vi "Periodic Tasks.vi"(8 "error in":errorcluster) -> ()   [LabVIEW 2014]
doc: "This VI runs in parallel to other tasks. It can contain as many user-defined periodic loops as you need. These can carry out PID or other sorts of timed response."
uses:
  <vilib>/Rock Robotics/WPI/Joystick/WPI_JoystickGetSetRefNum.vi
  Robot Global Data.vi
  <vilib>/Rock Robotics/Network Tables/SD Write Boolean.vi
  <vilib>/Rock Robotics/Network Tables/SD Write Number.vi
  <vilib>/Rock Robotics/WPI/RobotDrive/WPI_RobotDriveGetSetRefNum.vi
  <vilib>/Rock Robotics/WPI/Solenoid/WPI_SolenoidValue.ctl
  <vilib>/Rock Robotics/WPI/Solenoid/WPI_SolenoidSetEnum.vi
panel:
  in  "Stopper Motor Speed Up":dbl(slide)=0.6 min=-1.0 max=1.0 step=0.05 scale=0.0..1.0 scale format="%#.3f"
  in  "Stopper Motor Speed Down":dbl(slide)=0.2 min=-1.0 max=1.0 step=0.05 scale=0.0..1.0 scale format="%#.3f"
  out "Actual Stopper Motor Speed":dbl
  out "Lifting Motor Speed Up":dbl
  out "Mode":bool
  out "Actual Lifting Motor Speed":dbl format="%#_13g"
  out "Trigger Switch Activated":bool=TRUE
  out "Upper Switch Activated":bool=TRUE
  out "Lower Switch Activated":bool=TRUE
  out "Accelerometer Chart":cluster{"X-Axis":dbl, "Y-Axis":dbl}(graph)
  out "X Acceleration":dbl format="%#_13g"
  out "Y Acceleration":dbl format="%#_13g"
  out "Degrees of Rotation":dbl format="%#_13g"
  out "pnumatics button":bool
  out "L":bool
  out "U":bool
  out "T":bool
  out "Running":bool
  out "Direction":bool
  in  "Lifting Motor Speed Down":dbl(slide)=0.2 min=-1.0 max=1.0 step=0.05 scale=0.0..1.0 scale format="%#.3f"
  # "STOPPER\nMOTOR PANEL"
  # "GANTRY LIFT\nMOTOR PANEL"
  # "INDICATORS"
  # "LOGIC"
  # "CONTROLS"
  # "CONTROLS"
  # "INDICATORS"
  # "ACCELEROMETER\nPANEL"
  # "PNEUMATICS\nPANEL"
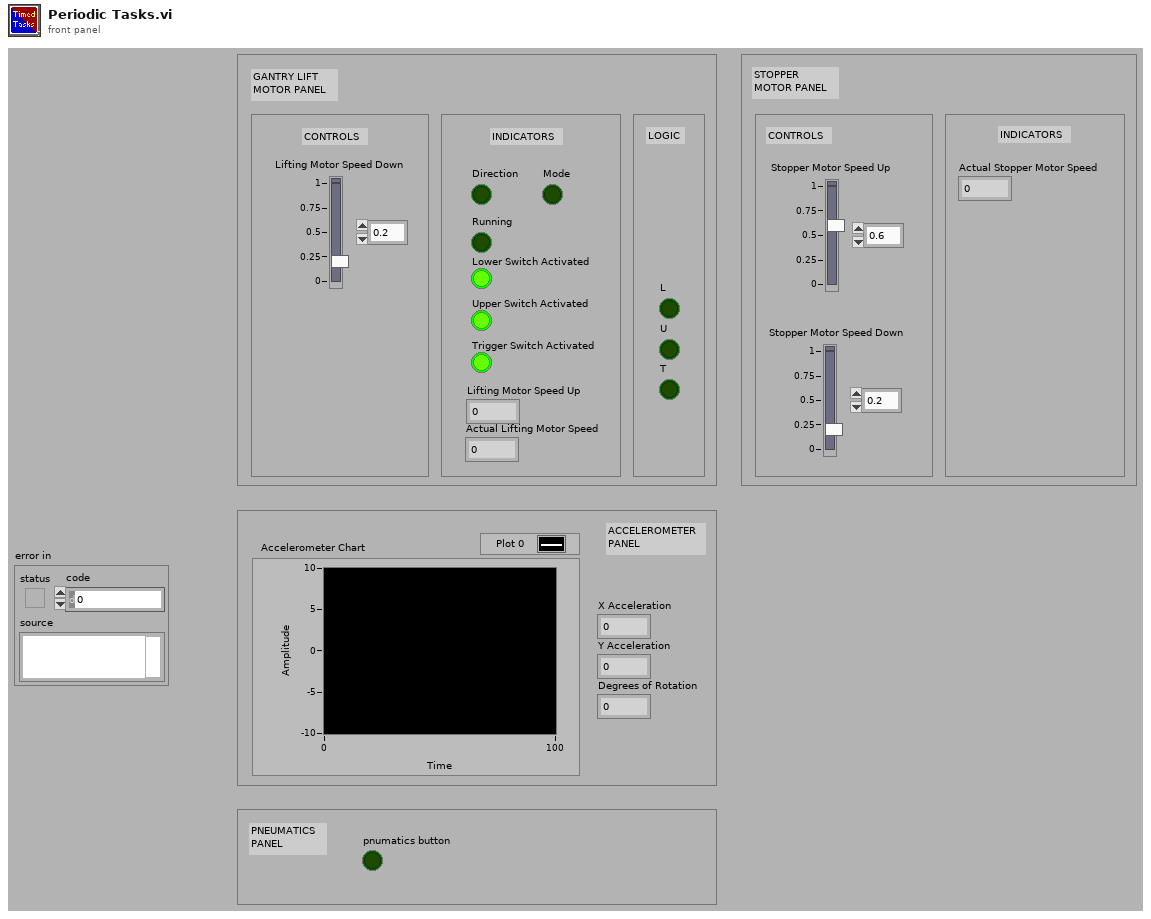
[diagram p1: front panel]
types:
  T1 = typedef "WPI_SolenoidValue.ctl" = enum16{"Off", "On", "Forward", "Reverse"}
  T2 = typedef "WPI_JoystickDevRef.ctl" = cluster{"Device":T3}
  T3 = typedef "WPI_JoystickDeviceEnum.ctl" = enum16{"USB 0", "USB 1", "USB 2", "USB 3", "USB 4", "USB 5"}
  T4 = typedef "WPI_SolenoidDevRef.ctl" = cluster{"DevStatus":errorcluster, "Pneumatics Control Module":u8, "Forward Solenoid Channel":T5, "Reverse Solenoid Channel":T5}
  T5 = typedef "WPI_SolenoidChannel.ctl" = enum8{"Solenoid 0", "Solenoid 1", "Solenoid 2", "Solenoid 3", "Solenoid 4", "Solenoid 5", "Solenoid 6", "Solenoid 7", "Invalid"}
  T6 = cluster{"JoystickDevRef":T2, "SolenoidDevRef":T4}
  T7 = typedef "WPI_AccelerometerDevRef.ctl" = cluster{"DevStatus":errorcluster, "Controller":T8, "Scaling":T9, "Analog Channels":T10, "I2C Bus":T12, "SPI Bus":T13, "Accel Range":T14, "ADXL345 Axes":T15, "Handle":i32, "Device Address":u8, "Accel Type":enum16{"Analog", "ADXL345 I2C", "ADXL345 SPI", "Internal"}}
  T8 = typedef "FPGA_TypedefAnalogModule.ctl" = enum16{"Controller 1"}
  T9 = typedef "WPI_AccelerometerScaling.ctl" = cluster{"Gain (VoltsPerG)":dbl, "Center Voltage":dbl}
  T10 = typedef "WPI_AccelerometerAnalogChannels.ctl" = cluster{"X-Axis":T11, "Y-Axis":T11, "Z-Axis":T11}
  T11 = typedef "FPGA_AIChannel.ctl" = enum8{"AI 0", "AI 1", "AI 2", "AI 3", "AI MXP 0", "AI MXP 1", "AI MXP 2", "AI MXP 3", "Invalid"}
  T12 = typedef "i2c_bus.ctl" = enum16{"I2C On-Board", "I2C MXP", "Invalid"}
  T13 = typedef "spi_bus.ctl" = enum16{"SPI On-Board, CS0", "SPI On-Board, CS1", "SPI On-Board, CS2", "SPI On-Board, CS3", "SPI MXP", "Invalid"}
  T14 = typedef "ADXL345 Range.ctl" = u8
  T15 = typedef "WPI_AccelerometerADXL345 Axes.ctl" = cluster{"X-Axis":bool, "Y-Axis":bool, "Z-Axis":bool}
  T16 = cluster{"X-Axis":dbl, "Y-Axis":dbl, "Z-Axis":dbl}
  T17 = typedef "WPI_MotorControlDeviceRef.ctl" = cluster{"DeviceStatus":errorcluster, "Type":T18, "PWM":cluster{"Controller":T19, "PWM Channel":T20, "DeadBand":T21}, "CAN":cluster{"Device Number":u8, "Control Mode":T22, "Semaphore":T23, "Max Vout":dbl, "TalonSRX Control Mode":T24}, "Invert":bool, "TransformRef":T25, "InvTransformRef":T25}
  T18 = typedef "WPI_MotorControlType.ctl" = enum16{"PWM", "CAN", "CANTalonSRX"}
  T19 = typedef "FPGA_TypedefDigitalModule.ctl" = enum16{"Controller 1"}
  T20 = typedef "FPGA_DIOPWMChannel.ctl" = enum8{"PWM 0", "PWM 1", "PWM 2", "PWM 3", "PWM 4", "PWM 5", "PWM 6", "PWM 7", "PWM 8", "PWM 9", "PWM MXP 0", "PWM MXP 1", "PWM MXP 2", "PWM MXP 3", "PWM MXP 4", "PWM MXP 5", "PWM MXP 6", "PWM MXP 7", "PWM MXP 8", "PWM MXP 9", "Invalid"}
  T21 = typedef "WPI_PWMDeadband.ctl" = cluster{"Name":string, "maxPositivePwm":i32, "minPositivePwm":i32, "centerPwm":i32, "maxNegativePwm":i32, "minNegativePwm":i32, "angularRange":u16}
  T22 = typedef "WPI_CANJaguar_ControlMode.ctl" = enum8{"Percent VBus", "Current", "Speed", "Position", "Voltage"}
  T23 = typedef "Semaphore RefNum" = refnum<k1>
  T24 = typedef "WPI_CANTalonSRX_APIControlMode.ctl" = enum8{"Percent VBus", "Speed", "Position", "Slave", "Unchanged / Invalid"}
  T25 = typedef "WPI_PWMTransform_ConPane.ctl" = refnum<vi>
  T26 = typedef "WPI_DigitalInputDevRef.ctl" = cluster{"DevStatus":errorcluster, "DIO Channel":T27, "Controller":T19}
  T27 = typedef "FPGA_DIOChannel.ctl" = enum8{"DIO 0", "DIO 1", "DIO 2", "DIO 3", "DIO 4", "DIO 5", "DIO 6", "DIO 7", "DIO 8", "DIO 9", "DIO MXP 0", "DIO MXP 1", "DIO MXP 2", "DIO MXP 3", "DIO MXP 4", "DIO MXP 5", "DIO MXP 6", "DIO MXP 7", "DIO MXP 8", "DIO MXP 9", "DIO MXP 10", "DIO MXP 11", "DIO MXP 12", "DIO MXP 13", "DIO MXP 14", "DIO MXP 15", "Invalid"}
  T28 = cluster{"JoystickDevRef":T2, "MotorControlDevRef":T17}
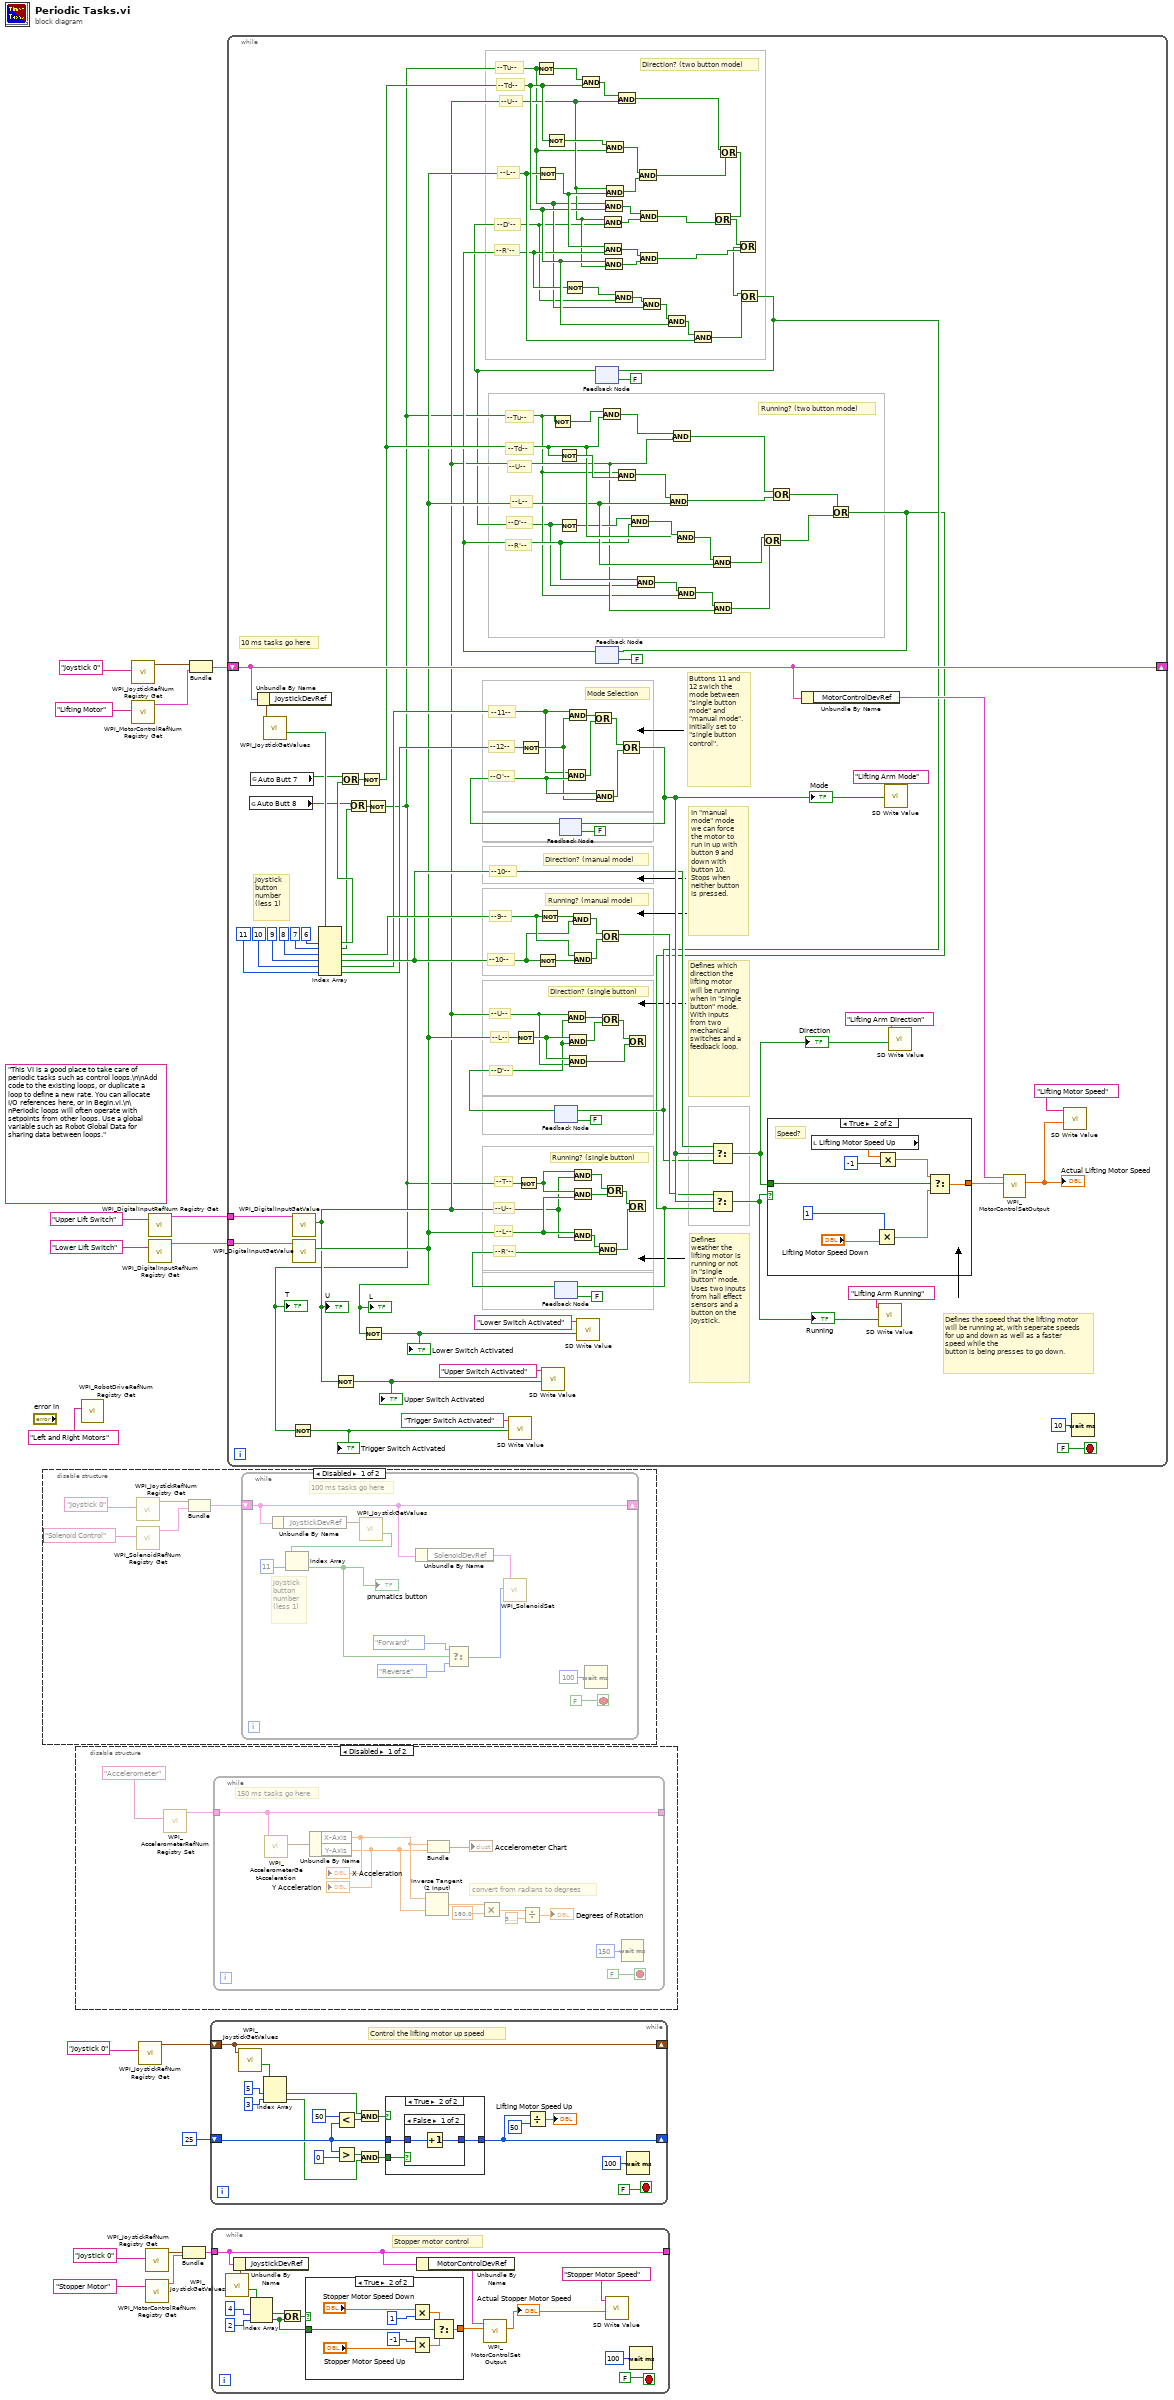
[diagram p0: block diagram]
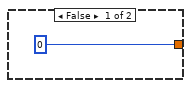
[diagram p2: hidden frame]
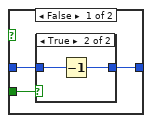
[diagram p3: hidden frame]
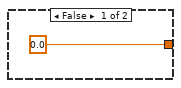
[diagram p8: hidden frame]
diagram:
  (unwired) "This VI is a good place to take care of periodic tasks such as control loops.\n\nAdd code to the existing loops, or duplicate a loop to define a new rate. You can allocate I/O references here, or in Begin.vi.\n\nPeriodic loops will often operate with setpoints from other loops. Use a global variable such as Robot Global Data for sharing data between loops."
  n1 = disable-structure shown="Disabled" {
    frame Disabled {
      n2 = call <vilib>:"WPI_JoystickRefNum Registry Get.vi"("refnum name"="Joystick 0") -> ("JoystickDevRef"=w21:T2)  [unwired: 1 in, 9 out]
      n3 = call <vilib>:"WPI_SolenoidRefNum Registry Get.vi"("refnum name"="Solenoid Control") -> ("SolenoidDevRef"=w20:T4)  [unwired: 9 in, 1 out]
      n4 = Bundle("JoystickDevRef"=w21, "SolenoidDevRef"=w20) -> (w19:T6)  [unwired: 1 out]
      n5 = while {
        shift-right: [w29] -> _
        shift-left: w19 -> [w29]
        stop <- FALSE stop-if-true
        # "Joystick button number (less 1)"
        # "100 ms tasks go here"
        n6 = Unbundle By Name(w29) -> ("JoystickDevRef"=w32:T2)
        n7 = call <vilib>:"WPI_JoystickGetValues.vi"("JoystickDevRef"=w32) -> ("Buttons"=w31:bool[])  [unwired: 6 in, 4 out]
        n8 = Index Array(array=w31, index=11) -> (element=w27:bool)
        "pnumatics button" <- w27
        n9 = Unbundle By Name(w29) -> ("SolenoidDevRef"=w28:T4)
        n10 = Select(t=WPI_SolenoidValue."Forward" ("Relay Value"), s=w27, f=WPI_SolenoidValue."Reverse" ("Relay Value")) -> (s? t:f=w24:T1)
        n11 = call-poly <vilib>:"WPI_SolenoidSet.vi"("Value"=w24, "SolenoidDevRef"=w28) -> ()  [unwired: 8 in, 2 out]
        n12 = Wait (ms)(milliseconds to wait=u32 100) -> ()  [unwired: 1 out]
      }
    }
    frame Enabled {
    }
  }
  n13 = disable-structure shown="Disabled" {
    frame Disabled {
      n14 = call <vilib>:"WPI_AccelerometerRefNum Registry Set.vi"("refnum name"="Accelerometer") -> ("AccelerometerDevRef"=w35:T7)  [unwired: 9 in, 1 out]
      n15 = while {
        tunnel: [w46] -> _
        tunnel: w35 -> [w46]
        stop <- FALSE stop-if-true
        # "convert from radians to degrees"
        # "150 ms tasks go here"
        n16 = call <vilib>:"WPI_AccelerometerGetAcceleration.vi"("AccelerometerDevRef"=w46) -> ("Accelerations"=w41:T16)  [unwired: 8 in, 2 out]
        n17 = Unbundle By Name(w41) -> ("X-Axis"=w39:dbl, "Y-Axis"=w38:dbl)
        "X Acceleration" <- w39
        "Y Acceleration" <- w38
        n18 = Inverse Tangent (2 Input)(1:w38, 2:w39) -> (0:w42:dbl)
        n19 = Bundle("X-Axis"=w39, "Y-Axis"=w38) -> (→"Accelerometer Chart":cluster{"X-Axis":dbl, "Y-Axis":dbl})  [unwired: 1 in]
        n20 = Multiply(x=w42, y=180.0) -> (x*y=w44:dbl)
        n21 = Divide(x=w44, y=3.141592653589793) -> (x/y=→"Degrees of Rotation":dbl)
        n22 = Wait (ms)(milliseconds to wait=u32 150) -> ()  [unwired: 1 out]
      }
    }
    frame Enabled {
    }
  }
  n23 = call <vilib>:"WPI_RobotDriveRefNum Registry Get.vi"("refnum name"="Left and Right Motors") -> ()  [unwired: 1 in, 10 out]
  n24 = call <vilib>:"WPI_JoystickRefNum Registry Get.vi"("refnum name"="Joystick 0") -> ("JoystickDevRef"=w14:T2)  [unwired: 1 in, 9 out]
  n25 = call <vilib>:"WPI_MotorControlRefNum Registry Get.vi"("refnum name"="Lifting Motor") -> ("MotorControlDevRef"=w10:T17)  [unwired: 9 in, 1 out]
  n26 = call <vilib>:"WPI_JoystickRefNum Registry Get.vi"("refnum name"="Joystick 0") -> ("JoystickDevRef"=w1:T2)  [unwired: 1 in, 9 out]
  n27 = call <vilib>:"WPI_JoystickRefNum Registry Get.vi"("refnum name"="Joystick 0") -> ("JoystickDevRef"=w5:T2)  [unwired: 1 in, 9 out]
  n28 = call <vilib>:"WPI_MotorControlRefNum Registry Get.vi"("refnum name"="Stopper Motor") -> ("MotorControlDevRef"=w4:T17)  [unwired: 9 in, 1 out]
  n29 = call <vilib>:"WPI_DigitalInputRefNum Registry Get.vi"("refnum name"="Upper Lift Switch") -> ("DigitalInputDevRef"=w12:T26)  [unwired: 9 in, 1 out]
  n30 = call <vilib>:"WPI_DigitalInputRefNum Registry Get.vi"("refnum name"="Lower Lift Switch") -> ("DigitalInputDevRef"=w11:T26)  [unwired: 9 in, 1 out]
  n31 = Bundle("JoystickDevRef"=w5, "MotorControlDevRef"=w4) -> (w3:T28)  [unwired: 1 in]
  n32 = Bundle("JoystickDevRef"=w14, "MotorControlDevRef"=w10) -> (w17:T28)  [unwired: 1 out]
  n33 = while {
    shift-right: [w57] -> _
    shift-left: 25 -> [w58]
    shift-right: [w49] -> _
    shift-left: w1 -> [w49]
    stop <- FALSE stop-if-true
    # "Control the lifting motor up speed"
    n34 = call <vilib>:"WPI_JoystickGetValues.vi"("JoystickDevRef"=w49) -> ("Buttons"=w55:bool[])  [unwired: 6 in, 4 out]
    n35 = Index Array(array=w55, index #1=5, index #2=3) -> (element #1=w52:bool, element #2=w51:bool)
    n36 = Less?(x=50, y=w58) -> (x < y?=w62:bool)
    n37 = Greater?(x=w58, y=0) -> (0:w61:bool)
    n38 = And(x=w52, y=w62) -> (x .and. y?=w60:bool)
    n39 = And(x=w61, y=w51) -> (x .and. y?=w59:bool)
    n40 = case shown="True" w60 {
      tunnel: w59 -> [w69 w75]
      tunnel: w58 -> [w68 w74]
      tunnel: [w67 w73] -> w57
      frame False {
        n41 = case shown="True" w69 {
          tunnel: w68 -> [w70 w72]
          tunnel: [w70 w71] -> w67
          frame False {
          }
          frame True {
            n42 = Decrement(x=w72) -> (x-1=w71:i32)
          }
        }
      }
      frame True {
        n43 = case shown="False" w75 {
          tunnel: w74 -> [w77 w78]
          tunnel: [w76 w78] -> w73
          frame False {
            n44 = Increment(x=w77) -> (x+1=w76:i32)
          }
          frame True {
          }
        }
      }
    }
    n45 = Divide(x=w57, y=50) -> (x/y=→"Lifting Motor Speed Up":dbl)
    n46 = Wait (ms)(milliseconds to wait=u32 100) -> ()  [unwired: 1 out]
  }
  n47 = while {
    tunnel: w3 -> [w83]
    tunnel: [w83] -> _
    stop <- FALSE stop-if-true
    # "Stopper motor control"
    n48 = Unbundle By Name(w83) -> ("JoystickDevRef"=w84:T2)
    n49 = call <vilib>:"WPI_JoystickGetValues.vi"("JoystickDevRef"=w84) -> ("Buttons"=w90:bool[])  [unwired: 6 in, 4 out]
    n50 = Index Array(array=w90, index #1=4, index #2=2) -> (element #1=w87:bool, element #2=w85:bool)
    n51 = Or(x=w87, y=w85) -> (x .or. y?=w86:bool)
    n52 = case shown="True" w86 {
      tunnel: w85 -> [_ w101]
      tunnel: [0 w99] -> w81
      frame False {
      }
      frame True {
        n53 = Multiply(x="Stopper Motor Speed Down", y=1) -> (x*y=w100:dbl)
        n54 = Multiply(x=-1, y="Stopper Motor Speed Up") -> (x*y=w96:dbl)
        n55 = Select(t=w100, s=w101, f=w96) -> (s? t:f=w99:dbl)
      }
    }
    n56 = Unbundle By Name(w83) -> ("MotorControlDevRef"=w82:T17)
    n57 = call <vilib>:"WPI_MotorControlSetOutput.vi"("Output"=w81, "MotorControlDevRef"=w82) -> ("Motor Output"=w79:dbl)  [unwired: 7 in, 2 out]
    "Actual Stopper Motor Speed" <- w79
    n58 = call-poly <vilib>:"SD Write Value.vi"("Numeric"=w79, "Name"="Stopper Motor Speed" ("refnum name")) -> ()  [unwired: 8 in, 2 out]
    n59 = Wait (ms)(milliseconds to wait=u32 100) -> ()  [unwired: 1 out]
  }
  n60 = while {
    shift-right: [w208] -> _
    shift-left: w17 -> [w208]
    tunnel: w12 -> [w212]
    tunnel: w11 -> [w210]
    stop <- FALSE stop-if-true
    # "Running? (two button mode)"
    # "Direction? (two button mode)"
    # "--R'--"
    # "--D'--"
    # "--L--"
    # "--U--"
    # "--Td--"
    # "--Tu--"
    # "--D'--"
    # "--R'--"
    # "--L--"
    # "--U--"
    # "--Td--"
    # "--Tu--"
    # "--10--"
    # "Direction? (manual mode)"
    # "--R'--"
    # "Running? (manual mode)"
    # "--O'--"
    # "Defines the speed that the lifting motor will be running at, with seperate speeds for up and down as well as a faster speed while the \nbutton is being presses to go down."
    # "Defines weather the lifting motor is running or not in \"single button\" mode. Uses two inputs from hall effect sensors and a button on the joystick."
    # "Defines which direction the lifting motor will be running when in \"single button\" mode. With inputs from two mechanical switches and a feedback loop."
    # "In \"manual mode\" mode we can force the motor to run in up with button 9 and down with button 10. Stops when neither button is pressed."
    # "Buttons 11 and 12 swich the mode between  \"single button mode\" and \"manual mode\". Initially set to \"single button control\"."
    # "--12--"
    # "--11--"
    # "--10--"
    # "--9--"
    # "Mode Selection"
    # "Joystick button number (less 1)"
    # "--U--"
    # "--L--"
    # "--T--"
    # "--D'--"
    # "--U--"
    # "--L--"
    # "Direction? (single button)"
    # "Running? (single button)"
    # "10 ms tasks go here"
    n61 = global read "Robot Global Data.vi" "Auto Butt 8"() -> (w104:bool)
    n62 = global read "Robot Global Data.vi" "Auto Butt 7"() -> (w108:bool)
    n63 = Unbundle By Name(w208) -> ("JoystickDevRef"=w211:T2)
    n64 = call <vilib>:"WPI_JoystickGetValues.vi"("JoystickDevRef"=w211) -> ("Buttons"=w190:bool[])  [unwired: 6 in, 4 out]
    n65 = call <vilib>:"WPI_DigitalInputGetValue.vi"("DigitalInputDevRef"=w212) -> ("Value"=w120:bool)  [unwired: 8 in, 2 out]
    "U" <- w120
    n66 = call <vilib>:"WPI_DigitalInputGetValue.vi"("DigitalInputDevRef"=w210) -> ("Value"=w126:bool)  [unwired: 8 in, 2 out]
    "L" <- w126
    n67 = Index Array(array=w190, index #1=u32 6 ("milliseconds to wait"), index #2=u32 7 ("milliseconds to wait"), index #3=u32 8 ("milliseconds to wait"), index #4=u32 9 ("milliseconds to wait"), index #5=u32 10 ("milliseconds to wait"), index #6=u32 11 ("milliseconds to wait")) -> (element #1=w107:bool, element #2=w105:bool, element #3=w165:bool, element #4=w161:bool, element #5=w158:bool, element #6=w157:bool)
    n68 = Not(x=w120) -> (.not. x?=w197:bool)
    "Upper Switch Activated" <- w197
    n69 = Or(x=w108, y=w107) -> (x .or. y?=w106:bool)
    n70 = Or(x=w104, y=w105) -> (x .or. y?=w192:bool)
    n71 = Not(x=w106) -> (.not. x?=w128:bool)
    n72 = Not(x=w126) -> (.not. x?=w198:bool)
    "Lower Switch Activated" <- w198
    n73 = Not(x=w192) -> (.not. x?=w119:bool)
    "T" <- w119
    n74 = Not(x=w119) -> (.not. x?=w195:bool)
    "Trigger Switch Activated" <- w195
    n75 = call-poly <vilib>:"SD Write Value.vi"("Boolean"=w195, "Name"="Trigger Switch Activated" ("refnum name")) -> ()  [unwired: 8 in, 2 out]
    n76 = Not(x=w126) -> (.not. x?=w178:bool)
    n77 = Not(x=w119) -> (.not. x?=w181:bool)
    n78 = Not(x=w157) -> (.not. x?=w172:bool)
    n79 = Not(x=w119) -> (.not. x?=w155:bool)
    n80 = Not(x=w126) -> (.not. x?=w134:bool)
    n81 = Not(x=w161) -> (.not. x?=w166:bool)
    n82 = Not(x=w165) -> (.not. x?=w167:bool)
    n83 = call-poly <vilib>:"SD Write Value.vi"("Boolean"=w197, "Name"="Upper Switch Activated" ("refnum name")) -> ()  [unwired: 8 in, 2 out]
    n84 = Not(x=w128) -> (.not. x?=w152:bool)
    n85 = Not(x=w119) -> (.not. x?=w121:bool)
    n86 = feedback #1(FALSE) -> (w173:bool)
    n87 = feedback #2(FALSE) -> (w180:bool)
    n88 = Not(x=w128) -> (.not. x?=w130:bool)
    n89 = feedback #3(FALSE) -> (w185:bool)
    n90 = And(x=w158, y=w185) -> (x .and. y?=w188:bool)
    n91 = And(x=w120, y=w173) -> (x .and. y?=w176:bool)
    n92 = And(x=w158, y=w172) -> (x .and. y?=w189:bool)
    n93 = And(x=w178, y=w173) -> (x .and. y?=w175:bool)
    n94 = And(x=w178, y=w120) -> (x .and. y?=w174:bool)
    n95 = And(x=w167, y=w161) -> (x .and. y?=w164:bool)
    n96 = And(x=w165, y=w166) -> (x .and. y?=w163:bool)
    n97 = And(x=w181, y=w120) -> (x .and. y?=w203:bool)
    n98 = And(x=w181, y=w126) -> (x .and. y?=w202:bool)
    n99 = And(x=w126, y=w120) -> (x .and. y?=w182:bool)
    n100 = call-poly <vilib>:"SD Write Value.vi"("Boolean"=w198, "Name"="Lower Switch Activated" ("refnum name")) -> ()  [unwired: 8 in, 2 out]
    n101 = And(x=w155, y=w128) -> (x .and. y?=w153:bool)
    n102 = Or(x=w189, y=w188) -> (x .or. y?=w187:bool)
    n103 = And(x=w185, y=w172) -> (x .and. y?=w186:bool)
    n104 = feedback #4(FALSE) -> (w118:bool)
    n105 = Not(x=w118) -> (.not. x?=w122:bool)
    n106 = feedback #5(FALSE) -> (w123:bool)
    n107 = Not(x=w123) -> (.not. x?=w133:bool)
    n108 = And(x=w182, y=w180) -> (x .and. y?=w179:bool)
    n109 = Or(x=w164, y=w163) -> (x .or. y?=w162:bool)
    n110 = Or(x=w176, y=w175) -> (x .or. y?=w177:bool)
    n111 = And(x=w121, y=w128) -> (x .and. y?=w132:bool)
    n112 = And(x=w120, y=w118) -> (x .and. y?=w146:bool)
    n113 = And(x=w134, y=w123) -> (x .and. y?=w143:bool)
    n114 = And(x=w119, y=w128) -> (x .and. y?=w147:bool)
    n115 = And(x=w128, y=w120) -> (x .and. y?=w142:bool)
    n116 = And(x=w152, y=w119) -> (x .and. y?=w151:bool)
    n117 = And(x=w120, y=w134) -> (x .and. y?=w150:bool)
    n118 = Or(x=w203, y=w202) -> (x .or. y?=w201:bool)
    n119 = And(x=w133, y=w118) -> (x .and. y?=w139:bool)
    n120 = And(x=w153, y=w120) -> (x .and. y?=w111:bool)
    n121 = And(x=w119, y=w130) -> (x .and. y?=w131:bool)
    n122 = Or(x=w187, y=w186) -> (x .or. y?=w170:bool)
    "Mode" <- w170
    n123 = feedback-in #3(w170) -> ()
    n124 = Or(x=w177, y=w174) -> ()  [unwired: 1 out]
    n125 = Or(x=w201, y=w179) -> ()  [unwired: 1 out]
    n126 = And(x=w122, y=w123) -> (x .and. y?=w129:bool)
    n127 = And(x=w123, y=w118) -> (x .and. y?=w124:bool)
    n128 = And(x=w151, y=w150) -> (x .and. y?=w149:bool)
    n129 = And(x=w147, y=w146) -> (x .and. y?=w145:bool)
    n130 = And(x=w143, y=w142) -> (x .and. y?=w141:bool)
    n131 = And(x=w139, y=w119) -> (x .and. y?=w138:bool)
    n132 = And(x=w138, y=w128) -> (x .and. y?=w137:bool)
    n133 = And(x=w131, y=w126) -> (x .and. y?=w116:bool)
    n134 = And(x=w132, y=w120) -> (x .and. y?=w117:bool)
    n135 = And(x=w129, y=w128) -> (x .and. y?=w127:bool)
    n136 = And(x=w124, y=w119) -> (x .and. y?=w125:bool)
    n137 = And(x=w137, y=w126) -> (x .and. y?=w135:bool)
    n138 = And(x=w127, y=w126) -> (x .and. y?=w115:bool)
    n139 = And(x=w125, y=w120) -> (x .and. y?=w114:bool)
    n140 = Or(x=w111, y=w149) -> (x .or. y?=w156:bool)
    n141 = Or(x=w156, y=w145) -> (x .or. y?=w140:bool)
    n142 = Or(x=w140, y=w141) -> (x .or. y?=w136:bool)
    n143 = Or(x=w136, y=w135) -> (x .or. y?=w110:bool)
    n144 = feedback-in #1(w110) -> ()
    n145 = feedback-in #4(w110) -> ()
    n146 = Select(t=w161, s=w170, f=w110) -> (s? t:f=w169:bool)
    "Direction" <- w169
    n147 = Or(x=w115, y=w114) -> (x .or. y?=w112:bool)
    n148 = Or(x=w117, y=w116) -> (x .or. y?=w113:bool)
    n149 = Unbundle By Name(w208) -> ("MotorControlDevRef"=w207:T17)
    n150 = Or(x=w113, y=w112) -> (x .or. y?=w109:bool)
    n151 = feedback-in #2(w109) -> ()
    n152 = feedback-in #5(w109) -> ()
    n153 = Select(t=w162, s=w170, f=w109) -> (s? t:f=w168:bool)
    "Running" <- w168
    n154 = case shown="True" w168 {
      tunnel: w169 -> [_ w223]
      tunnel: [0.0 ("Throw Motor Speed (-1 to 1) 2") w222] -> w193
      frame False {
      }
      frame True {
        # "Speed?"
        n155 = local read "Lifting Motor Speed Up"() -> (w216:dbl)
        n156 = Multiply(x=1, y="Lifting Motor Speed Down") -> (x*y=w219:dbl)
        n157 = Multiply(x=w216, y=-1) -> (x*y=w220:dbl)
        n158 = Select(t=w220, s=w223, f=w219) -> (s? t:f=w222:dbl)
      }
    }
    n159 = call-poly <vilib>:"SD Write Value.vi"("Boolean"=w168, "Name"="Lifting Arm Running" ("refnum name")) -> ()  [unwired: 8 in, 2 out]
    n160 = call-poly <vilib>:"SD Write Value.vi"("Boolean"=w170, "Name"="Lifting Arm Mode" ("refnum name")) -> ()  [unwired: 8 in, 2 out]
    n161 = call-poly <vilib>:"SD Write Value.vi"("Boolean"=w169, "Name"="Lifting Arm Direction" ("refnum name")) -> ()  [unwired: 8 in, 2 out]
    n162 = call <vilib>:"WPI_MotorControlSetOutput.vi"("Output"=w193, "MotorControlDevRef"=w207) -> ("Motor Output"=w103:dbl)  [unwired: 7 in, 2 out]
    "Actual Lifting Motor Speed" <- w103
    n163 = call-poly <vilib>:"SD Write Value.vi"("Numeric"=w103, "Name"="Lifting Motor Speed" ("refnum name")) -> ()  [unwired: 8 in, 2 out]
    n164 = Wait (ms)(milliseconds to wait=u32 10) -> ()  [unwired: 1 out]
  }
